vi "Global prova in corso.vi"() -> ()   [LabVIEW 2019]
panel:
  out "Reset tutti i timer":bool
  out "timer on":bool
  out "Prova a freddo":bool
  out "Reset tempo prova":bool
  out "MISURA RES IN CORSO":bool
  out "prova in corso?":bool
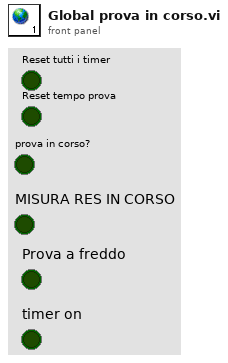
[diagram p1: front panel]
diagram:
